vi "Stop.vi"(8 "Error In":errorcluster) -> (0 "Error Out":errorcluster)   [LabVIEW 2017, in "Events.lvlib"]
uses:
  Events.lvlib
  Controls/Action Refs [enum].ctl
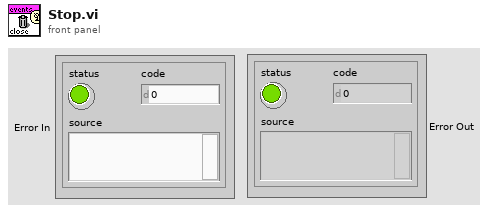
[diagram p1: front panel]
types:
  T1 = typedef "Events.lvlib/Action Refs [enum].ctl" = enum16{"Init", "Ref", "Kill"}
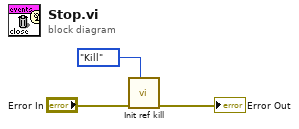
[diagram p0: block diagram]
diagram:
  n1 = call "Init ref kill.vi"("Action"=Action_Refs_[enum]."Kill", "Error In"="Error In") -> ("Error Out"=→"Error Out":errorcluster)  [unwired: 8 in, 1 out]
